vi "change table color.vi"(11 "MulticolumnListbox输入":refnum<vi>) -> ()   [LabVIEW 2016]
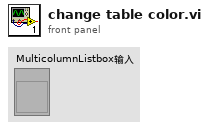
[diagram p1: front panel]
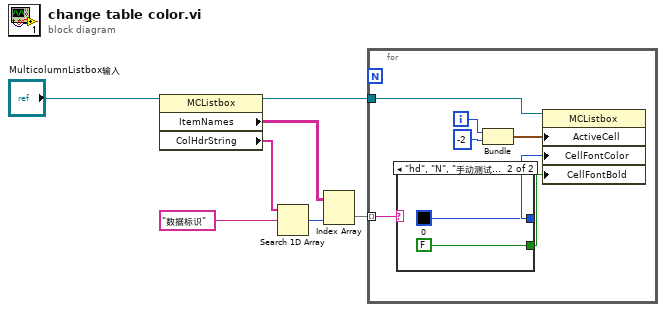
[diagram p0: block diagram]
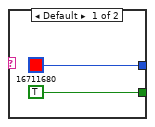
[diagram p2: hidden frame]
diagram:
  n1 = property class="MCListbox"(reference="MulticolumnListbox输入") -> (reference out=w7:refnum<vi>, "ItemNames"=w4:string[][], "ColHdrString"=w2:string[])  [unwired: 1 in, 1 out]
  n2 = Search 1D Array(1D array=w2, element="数据标识" ("元素")) -> (index of element=w5:i32)  [unwired: 1 in]
  n3 = Index Array(array=w4, index (col)=w5) -> (element=w6:string[])  [unwired: 1 in]
  n4 = for {
    tunnel: w6 -> [w14] mode=indexing
    tunnel: w7 -> [w13]
    i -> [w10]
    n5 = case shown="\"hd\", \"N\", \"手动测试数据\", \"正常数据\"" w14 {
      tunnel: [TRUE FALSE] -> w11
      tunnel: [u32 16711680 u32 0] -> w12
      frame Default {
      }
      frame "hd", "N", "手动测试数据", "正常数据" {
      }
    }
    n6 = Bundle(w10, -2) -> (w8:cluster{i32, i32})  [unwired: 1 in]
    n7 = property class="MCListbox"(reference=w13, "ActiveCell"=w8, "CellFontColor"=w12, "CellFontBold"=w11) -> ()  [unwired: 1 in, 2 out]
  }
